vi "DeleteDirALL.vi"(8 "error in (no error)":errorcluster, 10 "Path":path) -> (0 "error out":errorcluster)   [LabVIEW 2019, in "Tools.lvlib"]
uses:
  Tools.lvlib
panel:
  in  "application reference (local)":refnum<vi>
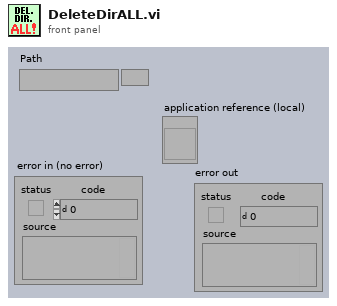
[diagram p1: front panel]
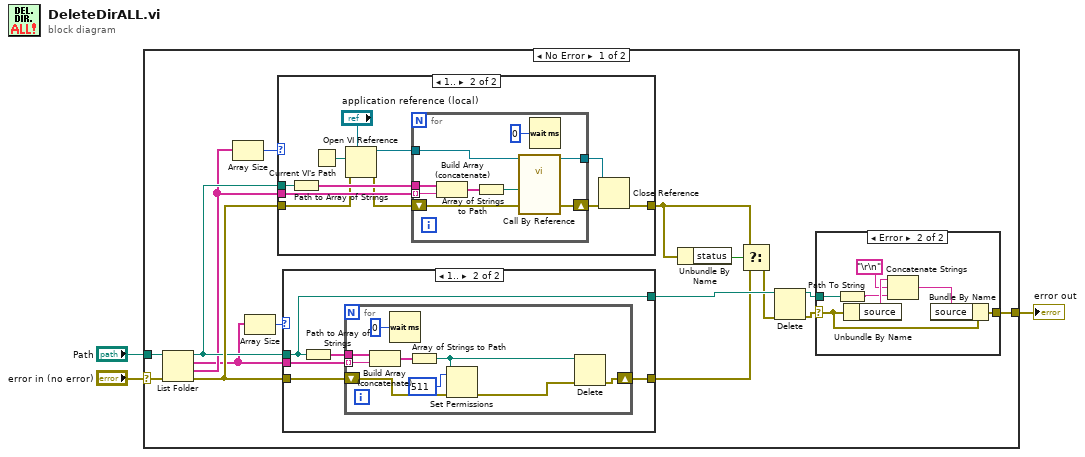
[diagram p0: block diagram]
diagram:
  n1 = case shown="No Error" "error in (no error)" {
    selector: "error in (no error)" -> [w19 w65]
    tunnel: [w11 w65] -> w2
    tunnel: "Path" -> [w18 _]
    frame No Error {
      n2 = List Folder(path=w18, error in=w19) -> (path out=w14:path, filenames=w8:string[], folder names=w9:string[], error out=w16:errorcluster)  [unwired: 2 in]
      n3 = Array Size(array=w9) -> (size(s)=w15:i32)
      n4 = Array Size(array=w8) -> (size(s)=w17:i32)
      n5 = case shown="1.." w15 {
        tunnel: w16 -> [w28 w36]
        tunnel: w14 -> [_ w38]
        tunnel: w9 -> [_ w39]
        tunnel: [w28 w30] -> w6
        frame 0, Default {
        }
        frame 1.. {
          n6 = Path to Array of Strings(0:w38) -> (2:w37:string[])  [unwired: 1 out]
          n7 = Current VI's Path() -> (path=w32:path)
          n8 = Open VI Reference(type specifier VI Refnum (for type only)="application reference (local)", vi path=w32, error in (no error)=w36) -> (vi reference=w33:refnum<vi>, error out=w35:errorcluster)  [unwired: 3 in]
          n9 = for {
            shift-right: [w43] -> w31
            shift-left: w35 -> [w44]
            tunnel: w39 -> [w48] mode=indexing
            tunnel: w37 -> [w47]
            tunnel: w33 -> [w41]
            tunnel: [w40] -> w29
            n10 = Build Array (concatenate)(w47, w48) -> (w46:string[])
            n11 = Array of Strings to Path(0:w46) -> (2:w42:path)  [unwired: 1 in]
            n12 = call-by-ref "?"(reference=w41, "error in (no error)"=w44, "Path"=w42) -> (reference out=w40:refnum<vi>, "error out"=w43:errorcluster)  [unwired: 10 in, 1 out]
            n13 = Wait (ms)(milliseconds to wait=u32 0) -> ()  [unwired: 1 out]
          }
          n14 = Close Reference(reference=w29, error in (no error)=w31) -> (error out=w30:errorcluster)
        }
      }
      n15 = case shown="1.." w17 {
        tunnel: w16 -> [w49 w55]
        tunnel: w14 -> [w50 w52]
        tunnel: w8 -> [_ w54]
        tunnel: [w50 w52] -> w13
        tunnel: [w49 w51] -> w5
        frame 0, Default {
        }
        frame 1.. {
          n16 = Path to Array of Strings(0:w52) -> (2:w53:string[])  [unwired: 1 out]
          n17 = for {
            shift-right: [w64] -> w51
            shift-left: w55 -> [w59]
            tunnel: w54 -> [w63] mode=indexing
            tunnel: w53 -> [w62]
            n18 = Build Array (concatenate)(w62, w63) -> (w61:string[])
            n19 = Wait (ms)(milliseconds to wait=u32 0) -> ()  [unwired: 1 out]
            n20 = Array of Strings to Path(0:w61) -> (2:w57:path)  [unwired: 1 in]
            n21 = Set Permissions(7:i16 511 ("new permissions"), 8:w59, 11:w57) -> (0:w58:errorcluster)  [unwired: 2 in, 1 out]
            n22 = Delete(path (use dialog)=w57, error in=w58) -> (error out=w64:errorcluster)  [unwired: 3 in, 2 out]
          }
        }
      }
      n23 = Unbundle By Name(w6) -> ("status"=w7:bool)
      n24 = Select(t=w6, s=w7, f=w5) -> (s? t:f=w4:errorcluster)
      n25 = Delete(path (use dialog)=w13, error in=w4) -> (deleted path=w10:path, error out=w12:errorcluster)  [unwired: 3 in, 1 out]
      n26 = case shown="Error" w12 {
        selector: w12 -> [w20 w26]
        tunnel: [w20 w27] -> w11
        tunnel: w10 -> [_ w25]
        frame No Error {
        }
        frame Error {
          n27 = Path To String(path=w25) -> (string=w23:string)
          n28 = Unbundle By Name(w26) -> ("source"=w24:string)
          n29 = Concatenate Strings(w24, "\r\n", w23) -> (w21:string)
          n30 = Bundle By Name(cluster=w26, "source"=w21) -> (w27:errorcluster)
        }
      }
    }
    frame Error {
    }
  }
  "error out" <- w2
